vi "HeaderAction.vi"(0 "InstrClass":refnum<class "AFG3102C.lvclass"> caption="DNL_LabVIEW Object in", 11 "error in (no error)":errorcluster caption="entrée d'erreur (pas d'erreur)") -> (4 "InstrClassOut":refnum<class "AFG3102C.lvclass"> caption="DNL_LabVIEW Object out", 6 "DataNames":string[](array[string]), 8 "Instr Name":string, 10 "HeaderString":string, 13 "ArrDisplayNames":string[](array[string]), 14 "DisplayNames":string[](array[string]), 15 "error out":errorcluster caption="sortie d'erreur")   [LabVIEW 2019, in "AFG3102C.lvclass"]
uses:
  AFG3102C.lvclass
  C:/Programmes Labview/LabScanV1A/DevicesClass/BaseDevice/BaseDevice.lvclass
  AFG3102C.lvclass/AFG3102C.ctl
  <userlib>/GenProg/ReadValByRefBool.vi
  <userlib>/GenProg/ReadValByRefDbl.vi
  BaseDevice/BaseDevice.lvclass
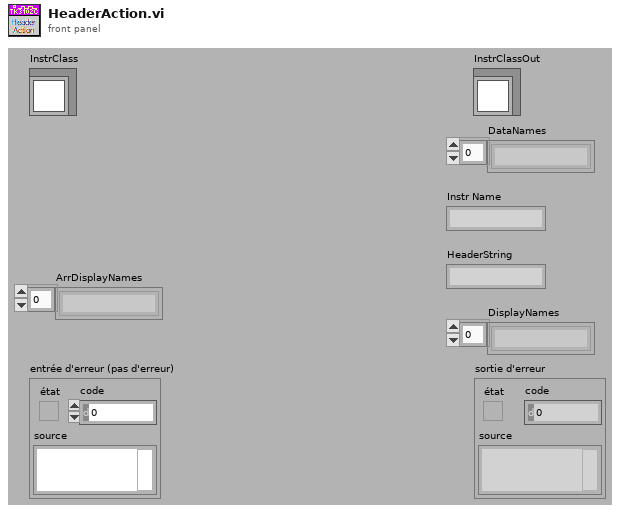
[diagram p1: front panel]
types:
  T1 = typedef "AFG3102C.lvclass/AFG3102C_Func.ctl" = enum16{"Rabi (Tau)", "Ramsey (Tau)"}
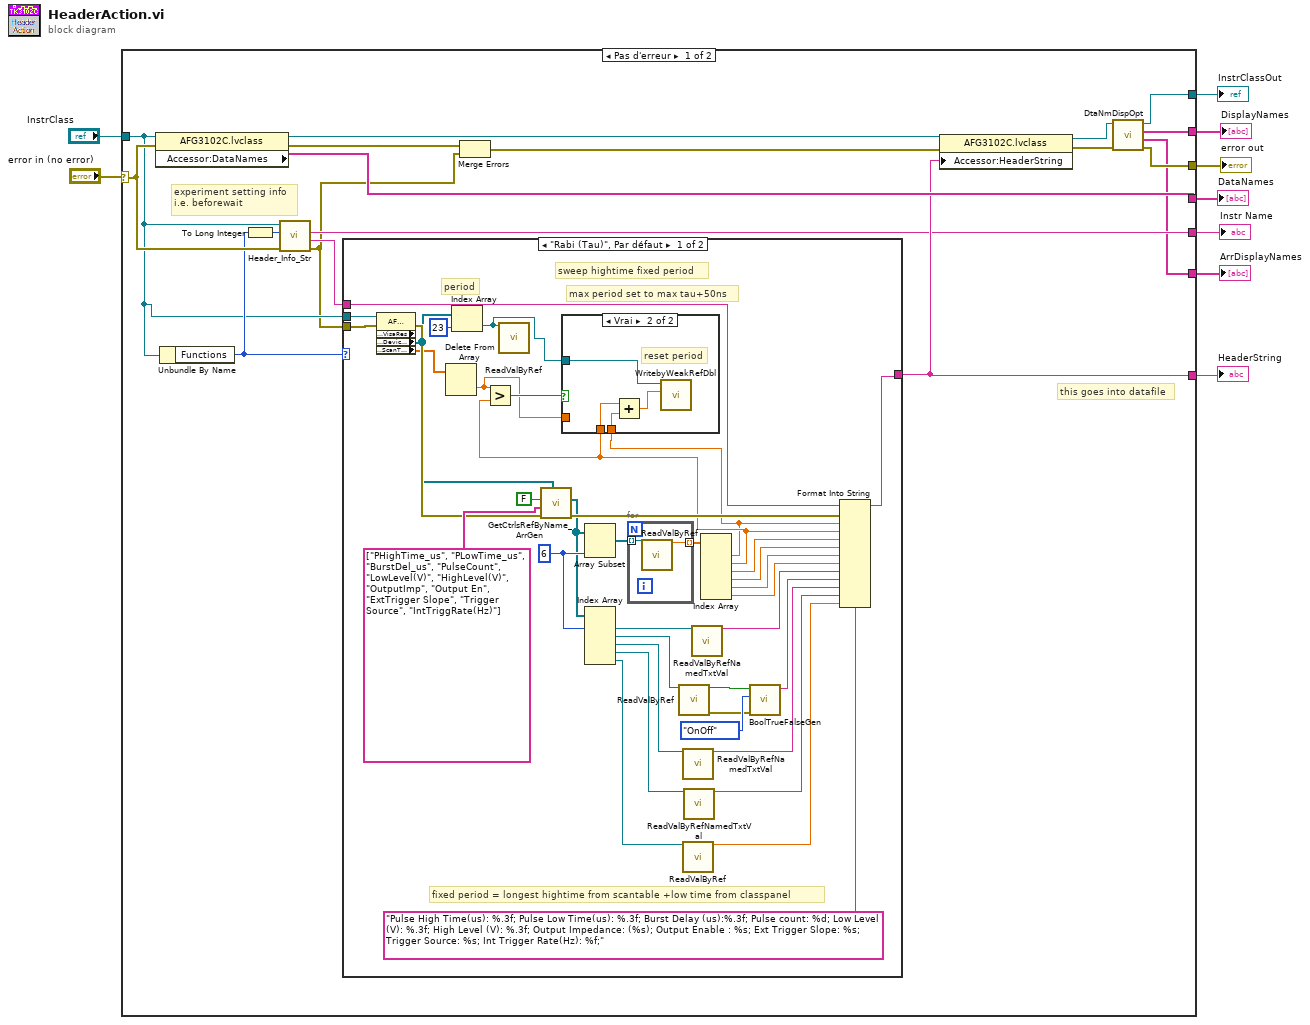
[diagram p0: block diagram]
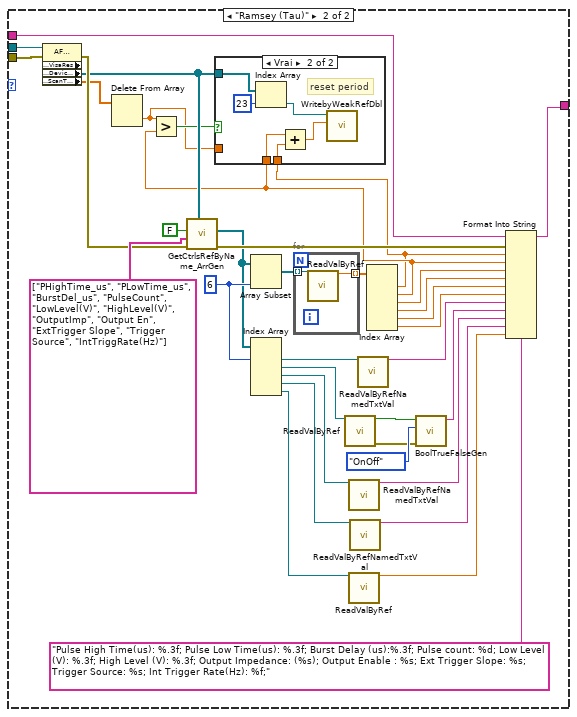
[diagram p3: hidden frame]
diagram:
  n1 = case shown="Pas d'erreur" "error in (no error)" {
    selector: "error in (no error)" -> [w16 w116]
    tunnel: [w24 _] -> w8
    tunnel: [w27 _] -> w7
    tunnel: "InstrClass" -> [w11 w117]
    tunnel: [w22 w116] -> w5
    tunnel: [w21 w117] -> w3
    tunnel: [w18 _] -> w4
    tunnel: [w19 _] -> w2
    tunnel: [w12 _] -> w1
    frame No Error {
      # "this goes into datafile"
      # "experiment setting info\ni.e. beforewait"
      n2 = property class="AFG3102C.lvclass"(reference=w11, error in=w16) -> (reference out=w26:refnum<class "AFG3102C.lvclass">, error out=w25:errorcluster, "Accessor:DataNames"=w27:string[])
      n3 = Unbundle By Name(w11) -> ("Functions"=w14:T1)
      n4 = To Long Integer(number=w14) -> (32bit integer=w13:i32)
      n5 = call-dynamic "Header_Info_Str.vi"("error in (no error)"=w16, "Functions"=w13, "DefaultDev in"=w11) -> ("error out"=w10:errorcluster, "HdrInfoStr"=w17:string, "InstrumentName"=w18:string)  [unwired: 5 in, 1 out]
      n6 = case shown="\"Rabi (Tau)\", Par défaut" w14 {
        tunnel: [w59 w101] -> w24
        tunnel: w17 -> [w60 w102]
        tunnel: w11 -> [w64 w106]
        tunnel: w10 -> [w63 w105]
        frame "Rabi (Tau)", Default {
          w46 = 6 ("longueur")
          # "fixed period = longest hightime from scantable +low time from classpanel"
          # "period"
          # "max period set to max tau+50ns"
          # "sweep hightime fixed period"
          n7 = property class="AFG3102C.lvclass" props=["Accessor:VisaRes", "Accessor:DeviceCtrl", "Accessor:ScanTable"](reference=w64, error in=w63) -> (error out=w57:errorcluster, "Accessor:DeviceCtrl"=w34:refnum<vi>[], "Accessor:ScanTable"=w35:dbl[])  [unwired: 2 out]
          n8 = Delete From Array(array=w35) -> (deleted portion=w32:dbl)  [unwired: 2 in, 1 out]
          n9 = Index Array(array=w34, index=23 ("indice")) -> (element=w28:refnum<vi>)
          n10 = call-poly <userlib>:"ReadValByRef.vi"("Control Ref"=w28) -> ()  [unwired: 13 in, 2 out]
          n11 = call <userlib>:"GetCtrlsRefByName_ArrGen.vi"("Commandes []"=w34, "ErrorIn(No Error)"=w57, "ControlName"=string[] ["PHighTime_us", "PLowTime_us", "BurstDel_us", "PulseCount", "LowLevel(V)", "HighLevel(V)", "OutputImp", "Output En", "ExtTrigger Slope", "Trigger Source", "IntTriggRate(Hz)"], "InclTabCTrl"=FALSE) -> ("sortie d'erreur"=w58:errorcluster, "ControlsRefs"=w44:refnum<vi>[])  [unwired: 5 in, 1 out]
          n12 = Array Subset(array=w44, length=w46) -> (w56:refnum<vi>[])  [unwired: 1 in]
          n13 = Index Array(array=w44, index #1=w46) -> (element #1=w43:refnum<vi>, element #2=w45:refnum<vi>, element #3=w41:refnum<vi>, element #4=w38:refnum<vi>, element #5=w37:refnum<vi>)  [unwired: 4 in]
          n14 = for {
            tunnel: w56 -> [w71] mode=indexing
            tunnel: [w70] -> w55 mode=indexing
            n15 = call-poly <userlib>:"ReadValByRef.vi"("Control Ref"=w71) -> ("Valeur"=w70:dbl)  [unwired: 13 in, 1 out]
          }
          n16 = call-poly <userlib>:"ReadValByRef.vi"("Control Ref"=w45) -> ("Valeur"=w49:bool, "error out"=w48:errorcluster)  [unwired: 13 in]
          n17 = call <userlib>:"ReadValByRefNamedTxtVal.vi"("Control Ref"=w41) -> ("Valeur"=w40:string)  [unwired: 13 in, 1 out]
          n18 = call-poly <userlib>:"ReadValByRef.vi"("Control Ref"=w37) -> ("Valeur"=w36:dbl)  [unwired: 13 in, 1 out]
          n19 = call <userlib>:"ReadValByRefNamedTxtVal.vi"("Control Ref"=w38) -> ("Valeur"=w39:string)  [unwired: 13 in, 1 out]
          n20 = call <userlib>:"ReadValByRefNamedTxtVal.vi"("Control Ref"=w43) -> ("Valeur"=w42:string)  [unwired: 13 in, 1 out]
          n21 = Index Array(array=w55) -> (element #1=w30:dbl, element #2=w31:dbl, element #3=w54:dbl, element #4=w53:dbl, element #5=w52:dbl, element #6=w51:dbl)  [unwired: 6 in]
          n22 = Greater?(x=w32, y=w31) -> (0:w33:bool)
          n23 = case shown="Vrai" w33 {
            tunnel: w32 -> [_ _]
            tunnel: w31 -> [_ w69]
            tunnel: w30 -> [_ w68]
            tunnel: w28 -> [_ w66]
            frame False {
            }
            frame True {
              # "reset period"
              n24 = Add(x=w69, y=w68) -> (x+y=w67:dbl)
              n25 = call <userlib>:"WritebyWeakRefDbl.vi"("Valeur"=w67, "Control Ref"=w66) -> ()  [unwired: 9 in, 1 out]
            }
          }
          n26 = call <userlib>:"BoolTrueFalseGen.vi"("Error in"=w48, "Énum"=enum16{"TrueFalse", "YesNo", "OnOff"}."OnOff", "Bool"=w49) -> ("TrueFalse"=w47:string)  [unwired: 6 in, 1 out]
          n27 = Format Into String(format string="Pulse High Time(us): %.3f; Pulse Low Time(us): %.3f; Burst Delay (us):%.3f; Pulse count: %d; Low Level (V): %.3f; High Level (V): %.3f; Output Impedance: (%s); Output Enable : %s; Ext Trigger Slope: %s; Trigger Source: %s; Int Trigger Rate(Hz): %f;" ("chaîne de format"), initial string=w60, error in=w58, w30, w31, w54, w53, w52, w51, w42, w47, w40, w39, w36) -> (resulting string=w59:string)  [unwired: 1 out]
        }
        frame "Ramsey (Tau)" {
          w88 = 6 ("longueur")
          n28 = property class="AFG3102C.lvclass" props=["Accessor:VisaRes", "Accessor:DeviceCtrl", "Accessor:ScanTable"](reference=w106, error in=w105) -> (error out=w99:errorcluster, "Accessor:DeviceCtrl"=w76:refnum<vi>[], "Accessor:ScanTable"=w77:dbl[])  [unwired: 2 out]
          n29 = Delete From Array(array=w77) -> (deleted portion=w74:dbl)  [unwired: 2 in, 1 out]
          n30 = call <userlib>:"GetCtrlsRefByName_ArrGen.vi"("Commandes []"=w76, "ErrorIn(No Error)"=w99, "ControlName"=string[] ["PHighTime_us", "PLowTime_us", "BurstDel_us", "PulseCount", "LowLevel(V)", "HighLevel(V)", "OutputImp", "Output En", "ExtTrigger Slope", "Trigger Source", "IntTriggRate(Hz)"], "InclTabCTrl"=FALSE) -> ("sortie d'erreur"=w100:errorcluster, "ControlsRefs"=w86:refnum<vi>[])  [unwired: 5 in, 1 out]
          n31 = Array Subset(array=w86, length=w88) -> (w98:refnum<vi>[])  [unwired: 1 in]
          n32 = Index Array(array=w86, index #1=w88) -> (element #1=w85:refnum<vi>, element #2=w87:refnum<vi>, element #3=w83:refnum<vi>, element #4=w80:refnum<vi>, element #5=w79:refnum<vi>)  [unwired: 4 in]
          n33 = for {
            tunnel: w98 -> [w115] mode=indexing
            tunnel: [w114] -> w97 mode=indexing
            n34 = call-poly <userlib>:"ReadValByRef.vi"("Control Ref"=w115) -> ("Valeur"=w114:dbl)  [unwired: 13 in, 1 out]
          }
          n35 = call-poly <userlib>:"ReadValByRef.vi"("Control Ref"=w87) -> ("Valeur"=w91:bool, "error out"=w90:errorcluster)  [unwired: 13 in]
          n36 = call <userlib>:"ReadValByRefNamedTxtVal.vi"("Control Ref"=w83) -> ("Valeur"=w82:string)  [unwired: 13 in, 1 out]
          n37 = call-poly <userlib>:"ReadValByRef.vi"("Control Ref"=w79) -> ("Valeur"=w78:dbl)  [unwired: 13 in, 1 out]
          n38 = call <userlib>:"ReadValByRefNamedTxtVal.vi"("Control Ref"=w80) -> ("Valeur"=w81:string)  [unwired: 13 in, 1 out]
          n39 = call <userlib>:"ReadValByRefNamedTxtVal.vi"("Control Ref"=w85) -> ("Valeur"=w84:string)  [unwired: 13 in, 1 out]
          n40 = Index Array(array=w97) -> (element #1=w72:dbl, element #2=w73:dbl, element #3=w96:dbl, element #4=w95:dbl, element #5=w94:dbl, element #6=w93:dbl)  [unwired: 6 in]
          n41 = Greater?(x=w74, y=w73) -> (0:w75:bool)
          n42 = case shown="Vrai" w75 {
            tunnel: w76 -> [_ w113]
            tunnel: w74 -> [_ _]
            tunnel: w73 -> [_ w110]
            tunnel: w72 -> [_ w109]
            frame False {
            }
            frame True {
              # "reset period"
              n43 = Index Array(array=w113, index=23 ("indice")) -> (element=w111:refnum<vi>)
              n44 = Add(x=w110, y=w109) -> (x+y=w108:dbl)
              n45 = call <userlib>:"WritebyWeakRefDbl.vi"("Valeur"=w108, "Control Ref"=w111) -> ()  [unwired: 9 in, 1 out]
            }
          }
          n46 = call <userlib>:"BoolTrueFalseGen.vi"("Error in"=w90, "Énum"=enum16{"TrueFalse", "YesNo", "OnOff"}."OnOff", "Bool"=w91) -> ("TrueFalse"=w89:string)  [unwired: 6 in, 1 out]
          n47 = Format Into String(format string="Pulse High Time(us): %.3f; Pulse Low Time(us): %.3f; Burst Delay (us):%.3f; Pulse count: %d; Low Level (V): %.3f; High Level (V): %.3f; Output Impedance: (%s); Output Enable : %s; Ext Trigger Slope: %s; Trigger Source: %s; Int Trigger Rate(Hz): %f;" ("chaîne de format"), initial string=w102, error in=w100, w72, w73, w96, w95, w94, w93, w84, w89, w82, w81, w78) -> (resulting string=w101:string)  [unwired: 1 out]
        }
      }
      n48 = Merge Errors(w25, w10) -> (w15:errorcluster)
      n49 = property class="AFG3102C.lvclass"(reference=w26, error in=w15, "Accessor:HeaderString"=w24) -> (reference out=w20:refnum<class "AFG3102C.lvclass">, error out=w23:errorcluster)
      n50 = call "DtaNmDispOpt.vi"("error in (no error)"=w23, "BaseDevice en entrée"=w20) -> ("error out"=w22:errorcluster, "ArrDisplayNames"=w12:string[], "DisplayNames"=w19:string[], "BaseDevice en sortie"=w21:refnum<class "AFG3102C.lvclass">)  [unwired: 6 in]
    }
    frame Error {
    }
  }
  "error out" <- w5
  "InstrClassOut" <- w3
  "DataNames" <- w7
  "HeaderString" <- w8
  "Instr Name" <- w4
  "DisplayNames" <- w2
  "ArrDisplayNames" <- w1
